vi "ReadAnInPan.vi"(8 "error in (no error)":errorcluster caption="entrée d'erreur (pas d'erreur)", 11 "EG_G5210.lvclass":refnum<class "EG_G5210.lvclass">) -> (0 "error out":errorcluster caption="sortie d'erreur", 3 "EG_G5210.lvclass Out":refnum<class "EG_G5210.lvclass">)   [LabVIEW 2010, in "EG_G5210.lvclass"]
uses:
  EG_G5210.lvclass
  BaseDevice/BaseDevice.lvclass
panel:
  out "Ch 4":dbl
  out "Ch 3":dbl
  out "Ch 2":dbl
  out "Ch 1":dbl
  in  "Stop":bool
  in  "MiseAJour":bool
  out "Init Program":bool
  # "EG&G 5210  Analog Inputs"
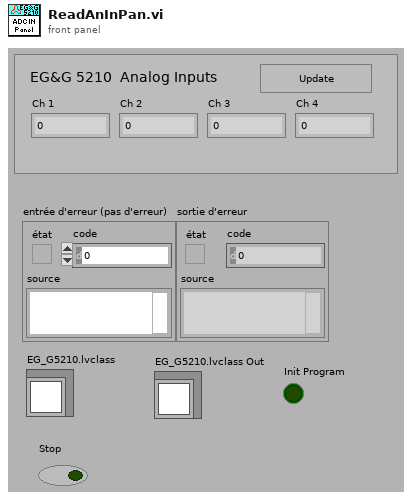
[diagram p1: front panel]
types:
  T1 = enum16{"X Output", "Y Output", "X and Y Output", "Mag", "Phase", "Mag & Phase", "X,Y,Mag & Phase", "Noise", "Aux In 1", "Aux In 2", "Aux In 3", "Aux In 4"}
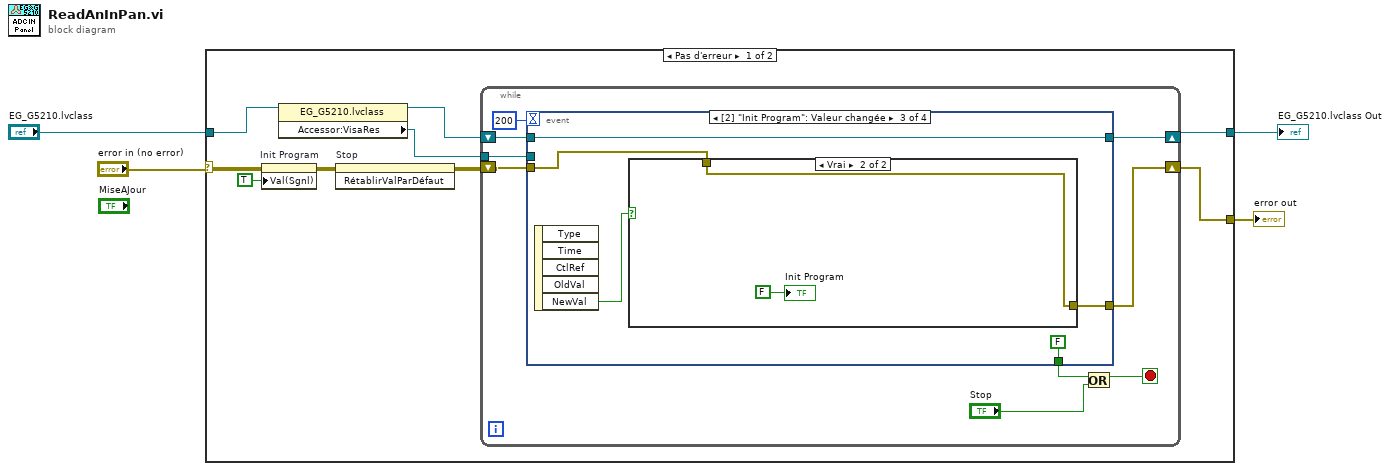
[diagram p0: block diagram]
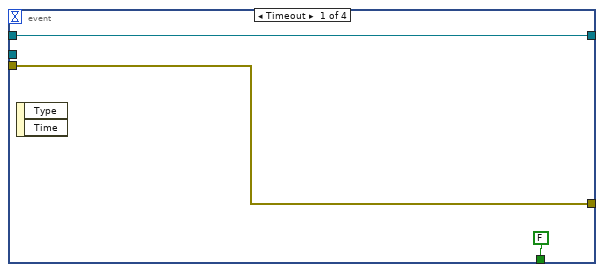
[diagram p2: hidden frame]
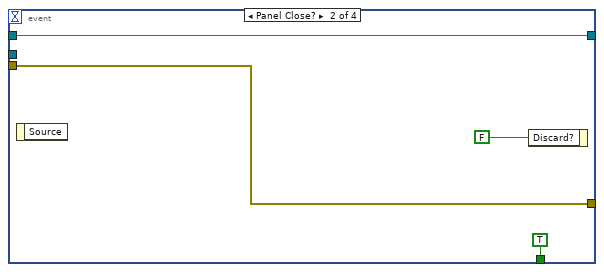
[diagram p3: hidden frame]
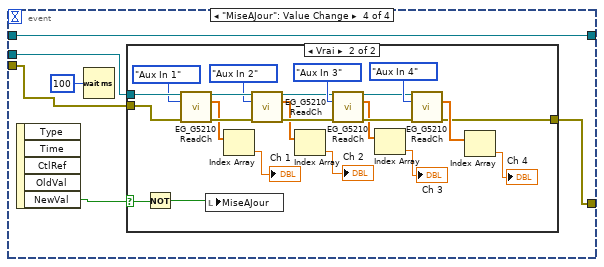
[diagram p5: hidden frame]
diagram:
  n1 = case shown="Pas d'erreur" "error in (no error)" {
    selector: "error in (no error)" -> [w10 w69]
    tunnel: [w13 w69] -> w3
    tunnel: "EG_G5210.lvclass" -> [w7 w68]
    tunnel: [w11 w68] -> w2
    frame No Error {
      n2 = property on="Init Program" class="Bool (strict)"(error in=w10, "Val(Sgnl)"=TRUE ("Valeur (Signalisation)")) -> (error out=w9:errorcluster)  [unwired: 1 in, 1 out]
      n3 = property class="EG_G5210.lvclass"(reference=w7) -> (reference out=w6:refnum<class "EG_G5210.lvclass">, "Accessor:VisaRes"=w5:refnum<visa-resource-name>)  [unwired: 1 in, 1 out]
      n4 = invoke on="Stop" class="Bool (strict)" method="RétablirValParDéfaut"(error in=w9) -> (error out=w8:errorcluster)  [unwired: 2 in, 2 out]
      n5 = while {
        shift-right: [w20] -> w13
        shift-left: w8 -> [w21]
        shift-right: [w17] -> w11
        shift-left: w6 -> [w19]
        tunnel: w5 -> [w14]
        stop <- w16 stop-if-true
        n6 = event shown="[2] \"Init Program\": Valeur changée" {
          selector: _ -> [_ _ _ _]
          dyn-events: _ -> [_ _ _ _]
          timeout: 200 -> [_ _ _ _]
          tunnel: w21 -> [w23 w27 w33 w39]
          tunnel: [w23 w27 w32 w38] -> w20
          tunnel: w19 -> [w24 w26 w31 w40]
          tunnel: [FALSE TRUE FALSE _] -> w18
          tunnel: [w24 w26 w31 w40] -> w17
          tunnel: w14 -> [_ _ _ w41]
          event Timeout {
            n7 = event-data() -> ()  [unwired: 1 in, 2 out]
          }
          event Panel Close? {
            n8 = event-data() -> ()  [unwired: 1 in, 1 out]
            n9 = event-data("Discard?"=FALSE ("Rejeter ?")) -> ()  [unwired: 1 in, 1 out]
          }
          event "Init Program": Value Change {
            n10 = event-data() -> ("NewVal"=w34:bool)  [unwired: 1 in, 4 out]
            n11 = case shown="Vrai" w34 {
              tunnel: w33 -> [w35 w36]
              tunnel: [w35 w36] -> w32
              frame False {
              }
              frame True {
                "Init Program" <- FALSE
              }
            }
          }
          event "MiseAJour": Value Change {
            n12 = event-data() -> ("NewVal"=w42:bool)  [unwired: 1 in, 4 out]
            n13 = Wait (ms)(milliseconds to wait=u32 100 ("attente (ms)")) -> ()  [unwired: 1 out]
            n14 = case shown="Vrai" w42 {
              selector: w42 -> [_ w67]
              tunnel: w41 -> [_ w65]
              tunnel: w39 -> [w44 w54]
              tunnel: [w44 w45] -> w38
              frame False {
              }
              frame True {
                n15 = Not(x=w67) -> (.not. x?=w66:bool)
                n16 = call <userlib>:"EG_G5210 ReadCh.vi"("VISA Rsrc"=w65, "Channel"=T1."Aux In 1", "error in (no error)"=w54) -> ("Ressource VISA Out"=w63:refnum<visa-resource-name>, "Outputs"=w52:dbl[], "error out"=w62:errorcluster)  [unwired: 5 in, 5 out]
                n17 = local write "MiseAJour"(w66) -> ()
                n18 = Index Array(array=w52) -> (element=→"Ch 1":dbl)  [unwired: 1 in]
                n19 = call <userlib>:"EG_G5210 ReadCh.vi"("VISA Rsrc"=w63, "Channel"=T1."Aux In 2", "error in (no error)"=w62) -> ("Ressource VISA Out"=w56:refnum<visa-resource-name>, "Outputs"=w49:dbl[], "error out"=w55:errorcluster)  [unwired: 5 in, 5 out]
                n20 = Index Array(array=w49) -> (element=→"Ch 2":dbl)  [unwired: 1 in]
                n21 = call <userlib>:"EG_G5210 ReadCh.vi"("VISA Rsrc"=w56, "Channel"=T1."Aux In 3", "error in (no error)"=w55) -> ("Ressource VISA Out"=w58:refnum<visa-resource-name>, "Outputs"=w48:dbl[], "error out"=w59:errorcluster)  [unwired: 5 in, 5 out]
                n22 = Index Array(array=w48) -> (element=→"Ch 3":dbl)  [unwired: 1 in]
                n23 = call <userlib>:"EG_G5210 ReadCh.vi"("VISA Rsrc"=w58, "Channel"=T1."Aux In 4", "error in (no error)"=w59) -> ("Outputs"=w53:dbl[], "error out"=w45:errorcluster)  [unwired: 5 in, 6 out]
                n24 = Index Array(array=w53) -> (element=→"Ch 4":dbl)  [unwired: 1 in]
              }
            }
          }
        }
        n25 = Or(x=w18, y="Stop") -> (x .or. y?=w16:bool)
      }
    }
    frame Error {
    }
  }
  "error out" <- w3
  "EG_G5210.lvclass Out" <- w2
